vi "save test.vi"() -> ()   [LabVIEW 2016]
uses:
  <vilib>/Utility/file.llb/Read Delimited Spreadsheet (DBL).vi
  <vilib>/Utility/file.llb/Write Delimited Spreadsheet (DBL).vi
panel:
  out "num2":dbl=-0.0
  out "appended array":dbl[][](array[numeric])
  in  "num test":bool
  in  "num1":i32=5
  out "appended path":path
  in  "t 3":dbl[][](array[numeric])
  in  "setting data 2":bool
  in  "t 2":dbl[][](array[numeric])
  out "s? t:f":dbl[][](array[numeric])
  in  "setting data":bool
  out "num2":dbl
  out "num1":dbl
  in  "t":dbl
  in  "Reference 2":bool
  in  "Reference":bool
  in  "save data1":bool
  in  "path":path=path "D:/Gantry_General/Main/ms_kao/gantry exericse/save test/001.txt"
  out "Array 2":dbl[](array[numeric])
  in  "Numeric":i32=5
  in  "stop":bool
  # "Reference test read value"
  # "set default file , read file value and save to file"
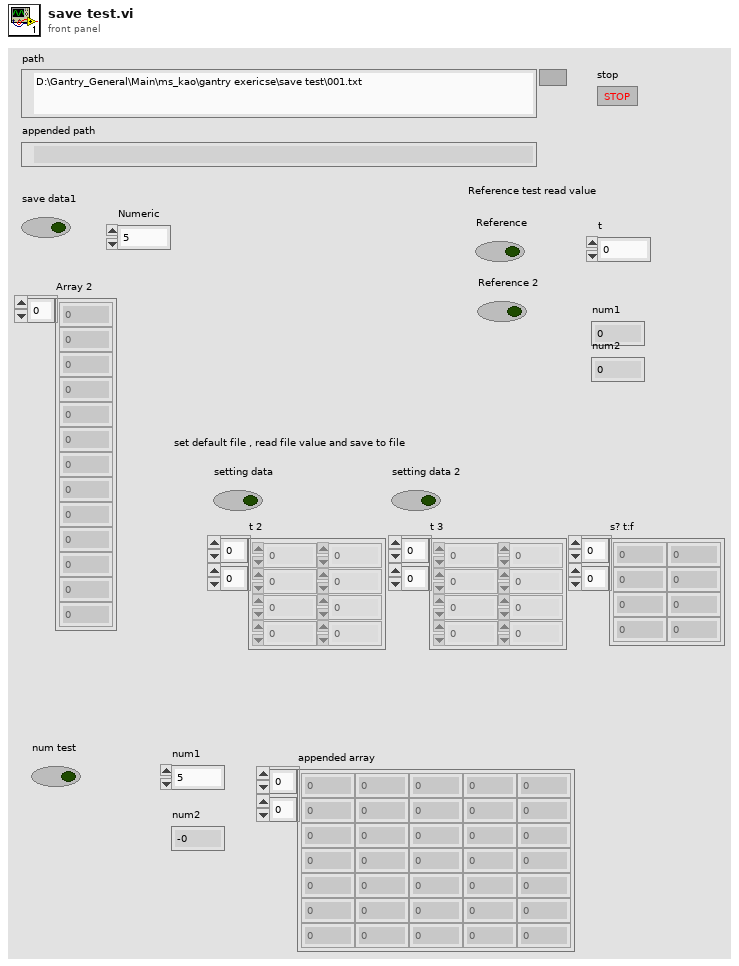
[diagram p1: front panel]
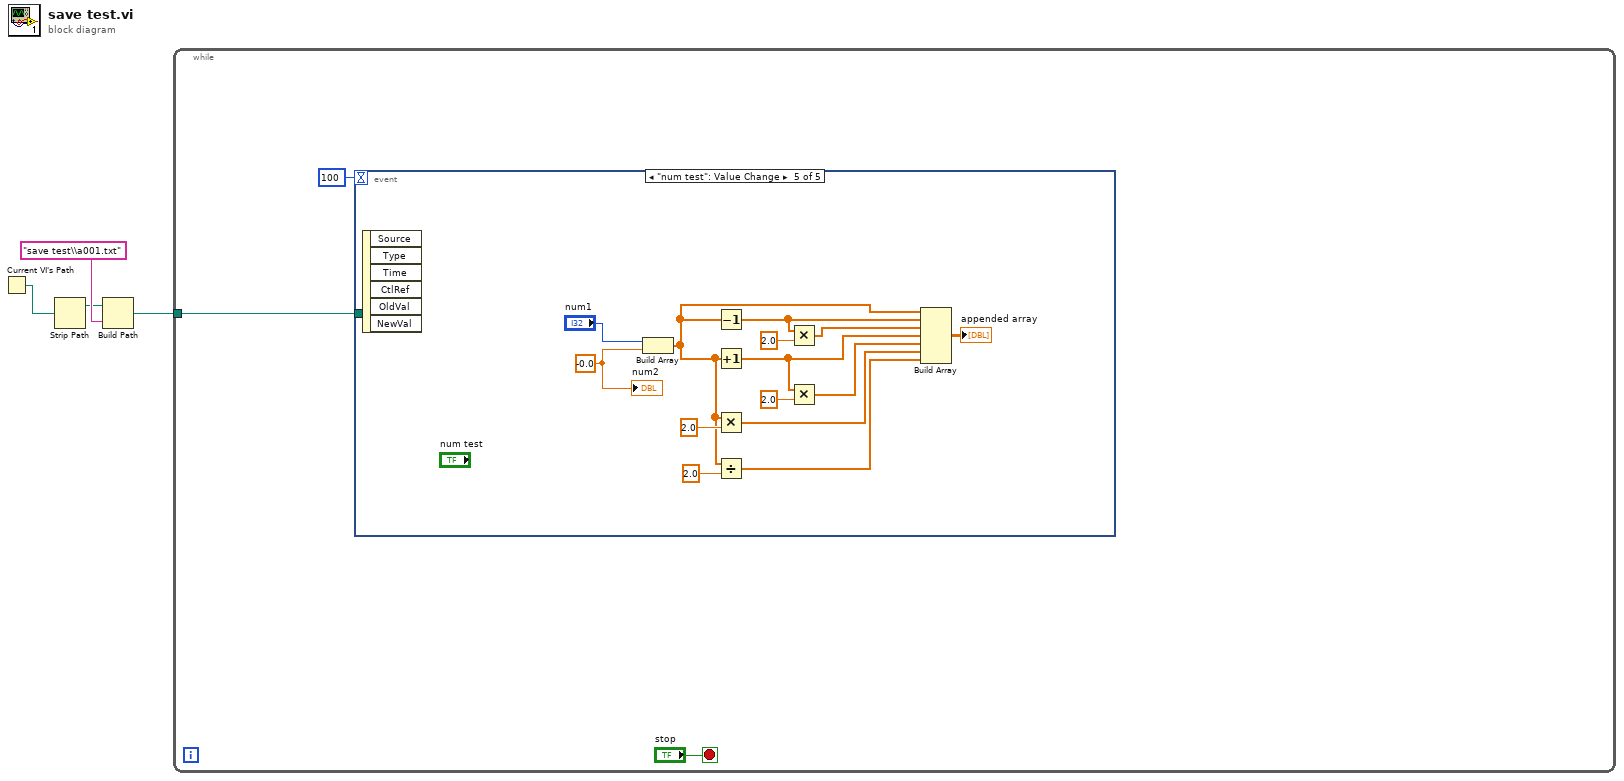
[diagram p0: block diagram]
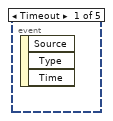
[diagram p2: hidden frame]
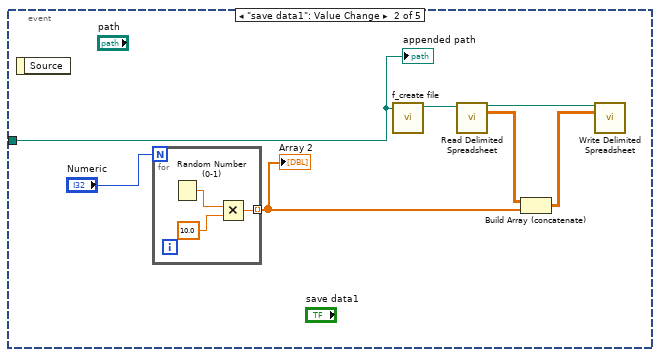
[diagram p3: hidden frame]
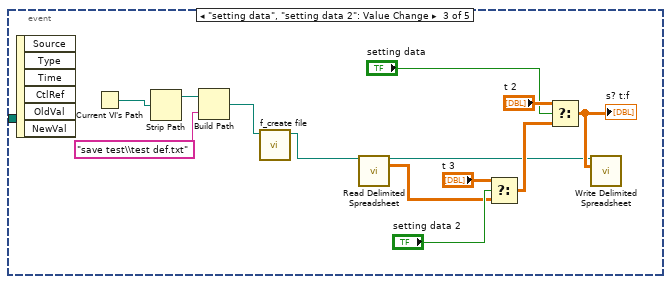
[diagram p4: hidden frame]
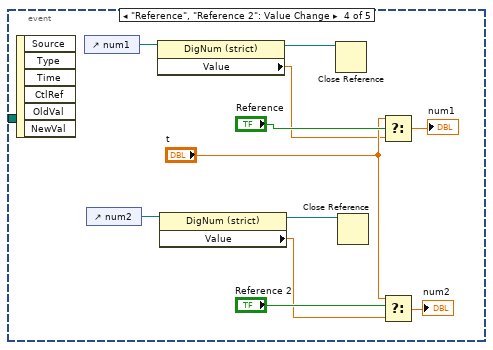
[diagram p5: hidden frame]
diagram:
  n1 = Current VI's Path() -> (path=w3:path)
  n2 = Strip Path(path=w3) -> (stripped path=w2:path)  [unwired: 1 out]
  n3 = Build Path(base path=w2, name or relative path="save test\\a001.txt") -> (appended path=w1:path)
  n4 = while {
    tunnel: w1 -> [w5]
    stop <- "stop" stop-if-true
    n5 = event shown="[4] \"num test\": Value Change" {
      selector: _ -> [_ _ _ _ _]
      dyn-events: _ -> [_ _ _ _ _]
      timeout: 100 -> [_ _ _ _ _]
      tunnel: w5 -> [_ w8 _ _ _]
      event Timeout {
        n6 = event-data() -> ()  [unwired: 1 in, 3 out]
      }
      event "save data1": Value Change {
        n7 = event-data() -> ()  [unwired: 1 in, 1 out]
        n8 = for {
          N: "Numeric" -> [_]
          tunnel: [w15] -> w9 mode=indexing
          n9 = Random Number (0-1)() -> (number: 0 to 1=w17:dbl)
          n10 = Multiply(x=w17, y=10.0) -> (x*y=w15:dbl)
        }
        "Array 2" <- w9
        n11 = call "f_create file.vi"("path"=w8) -> ("dup path"=w14:path)  [unwired: 10 in]
        n12 = call-poly <vilib>:"Read Delimited Spreadsheet.vi"("file path (dialog if empty)"=w14) -> ("new file path (Not A Path if cancelled)"=w12:path, "all rows"=w13:dbl[][])  [unwired: 9 in, 4 out]
        n13 = Build Array (concatenate)(w13, w9) -> (w11:dbl[][])
        n14 = call-poly <vilib>:"Write Delimited Spreadsheet.vi"("file path (dialog if empty)"=w12, "2D data"=w11) -> ()  [unwired: 12 in, 2 out]
        "appended path" <- w8
      }
      event "setting data", "setting data 2": Value Change {
        n15 = event-data() -> ()  [unwired: 1 in, 6 out]
        n16 = Current VI's Path() -> (path=w21:path)
        n17 = Strip Path(path=w21) -> (stripped path=w20:path)  [unwired: 1 out]
        n18 = Build Path(base path=w20, name or relative path="save test\\test def.txt") -> (appended path=w22:path)
        n19 = call "f_create file.vi"("path"=w22) -> ("dup path"=w18:path)  [unwired: 10 in]
        n20 = call-poly <vilib>:"Read Delimited Spreadsheet.vi"("file path (dialog if empty)"=w18) -> ("new file path (Not A Path if cancelled)"=w24:path, "all rows"=w23:dbl[][])  [unwired: 9 in, 4 out]
        n21 = Select(t="t 3", s="setting data 2", f=w23) -> (s? t:f=w28:dbl[][])
        n22 = Select(t="t 2", s="setting data", f=w28) -> (s? t:f=w25:dbl[][])
        "s? t:f" <- w25
        n23 = call-poly <vilib>:"Write Delimited Spreadsheet.vi"("file path (dialog if empty)"=w24, "2D data"=w25) -> ()  [unwired: 12 in, 2 out]
      }
      event "Reference", "Reference 2": Value Change {
        n24 = event-data() -> ()  [unwired: 1 in, 6 out]
        n25 = control-ref of="num1"() -> (w36:refnum<vi>)
        n26 = control-ref of="num2"() -> (w33:refnum<vi>)
        n27 = property class="DigNum (strict)"(reference=w36) -> (reference out=w35:refnum<vi>, "Value"=w31:dbl)  [unwired: 1 in, 1 out]
        n28 = property class="DigNum (strict)"(reference=w33) -> (reference out=w34:refnum<vi>, "Value"=w32:dbl)  [unwired: 1 in, 1 out]
        n29 = Close Reference(reference=w35) -> ()  [unwired: 1 in, 1 out]
        n30 = Close Reference(reference=w34) -> ()  [unwired: 1 in, 1 out]
        n31 = Select(t="t", s="Reference", f=w31) -> (s? t:f=→"num1":dbl)
        n32 = Select(t="t", s="Reference 2", f=w32) -> (s? t:f=→"num2":dbl)
      }
      event "num test": Value Change {
        w54 = -0.0
        n33 = event-data() -> ()  [unwired: 1 in, 6 out]
        n34 = Build Array("num1", w54) -> (w47:dbl[])
        n35 = Decrement(x=w47) -> (x-1=w49:dbl[])
        n36 = Increment(x=w47) -> (x+1=w46:dbl[])
        n37 = Multiply(x=w47, y=2.0) -> (x*y=w44:dbl[])
        n38 = Divide(x=w47, y=2.0) -> (x/y=w43:dbl[])
        n39 = Multiply(x=w49, y=2.0) -> (x*y=w48:dbl[])
        n40 = Multiply(x=w46, y=2.0) -> (x*y=w45:dbl[])
        n41 = Build Array(w47, w49, w48, w46, w45, w44, w43) -> (→"appended array":dbl[][])
        "num2" <- w54
      }
    }
  }
